vi "Add Default Free.vi"(8 "error in (no error)":errorcluster, 10 "ToModBus":bool, 11 "Frequency":refnum<class "Frequency.lvclass">) -> (0 "error out":errorcluster, 3 "Frequency Out":refnum<class "Frequency.lvclass">)   [LabVIEW 2018, in "Measurement Channels.lvlib" / "Frequency.lvclass"]
uses:
  Frequency.lvclass
  C:/Users/Jeff Tipps/Documents/DAQMan/source/Classes/Measurements/Class Channel/Channel.lvclass
  Frequency.lvclass/Frequency.ctl
  Class Channel/Write Unit_EU.vi
  Class Voltage/Voltage.lvclass
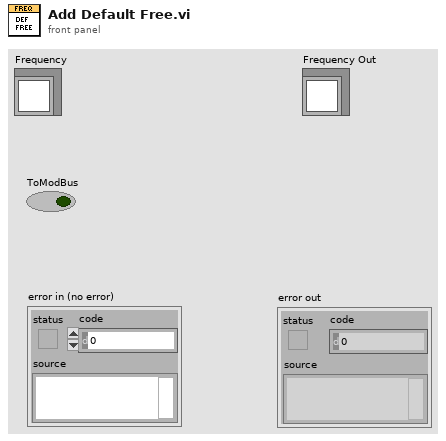
[diagram p1: front panel]
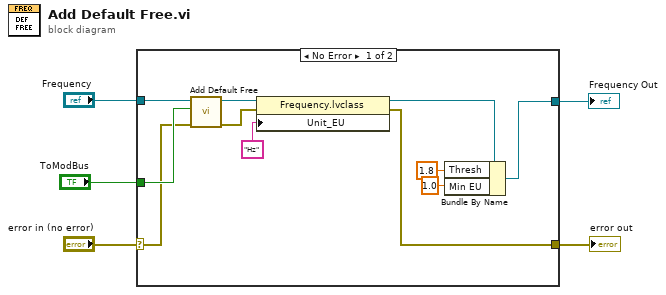
[diagram p0: block diagram]
diagram:
  n1 = case shown="No Error" "error in (no error)" {
    selector: "error in (no error)" -> [w11 w17]
    tunnel: "Frequency" -> [w13 w18]
    tunnel: [w6 w17] -> w5
    tunnel: [w16 w18] -> w4
    tunnel: "ToModBus" -> [w12 _]
    frame No Error {
      n2 = call-parent "Add Default Free.vi"("error in (no error)"=w11, "ToModBus"=w12, "Volt In"=w13) -> ("error out"=w9:errorcluster, "Volt Out"=w10:refnum<class "Frequency.lvclass">)  [unwired: 7 in]
      n3 = property class="Frequency.lvclass"(reference=w10, error in=w9, "Unit_EU"="Hz") -> (reference out=w7:refnum<class "Frequency.lvclass">, error out=w6:errorcluster)
      n4 = Bundle By Name(cluster=w7, "Thresh"=1.8, "Min EU"=1.0) -> (w16:refnum<class "Frequency.lvclass">)
    }
    frame Error {
    }
  }
  "Frequency Out" <- w4
  "error out" <- w5
